vi "Read User Visible Name.vi"(8 "error in (no error)":errorcluster, 11 "Client Proxy LNA in":refnum<class "Client Proxy LNA.lvclass">) -> (0 "error out":errorcluster, 2 "User Visible Name":string, 3 "Client Proxy LNA out":refnum<class "Client Proxy LNA.lvclass">)   [LabVIEW 2013, in "Client Proxy LNA.lvlib" / "Client Proxy LNA.lvclass"]
uses:
  Client Proxy LNA.lvclass
  Client Proxy LNA.lvclass/Client Proxy LNA.ctl
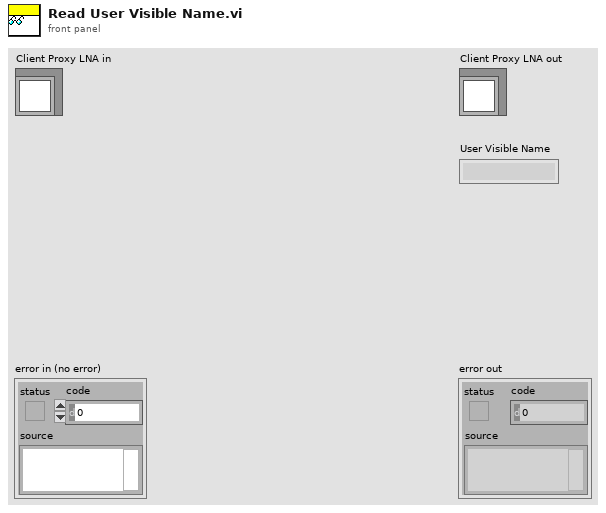
[diagram p1: front panel]
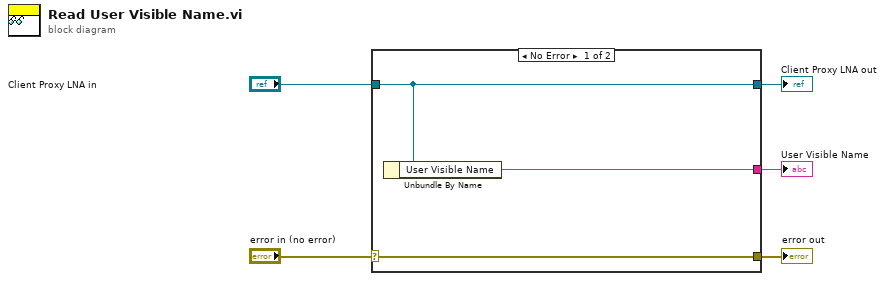
[diagram p0: block diagram]
diagram:
  n1 = case shown="No Error" "error in (no error)" {
    selector: "error in (no error)" -> [w8 w9]
    tunnel: [w8 w9] -> w4
    tunnel: [w7 w10] -> w2
    tunnel: "Client Proxy LNA in" -> [w7 w10]
    tunnel: [w6 _] -> w1
    frame No Error {
      n2 = Unbundle By Name(w7) -> ("User Visible Name"=w6:string)
    }
    frame Error {
    }
  }
  "error out" <- w4
  "Client Proxy LNA out" <- w2
  "User Visible Name" <- w1
